vi "CreateTerminalVoltageDAQTask.vi"(8 "Error In":errorcluster) -> (0 "Error Out":errorcluster, 3 "Terminal Voltage Task":refnum<k21>)   [LabVIEW 2012]
uses:
  <vilib>/DAQmx/create/channels.llb/DAQmx Create Channel (AI-Voltage-Basic).vi
  <vilib>/DAQmx/configure/timing.llb/DAQmx Timing (Sample Clock).vi
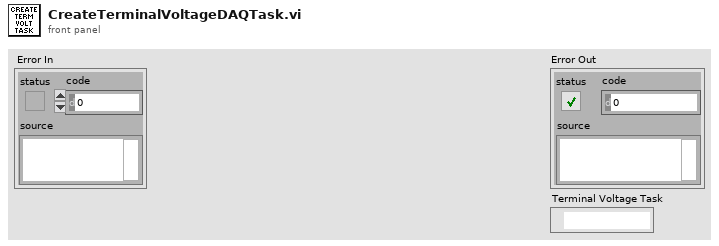
[diagram p1: front panel]
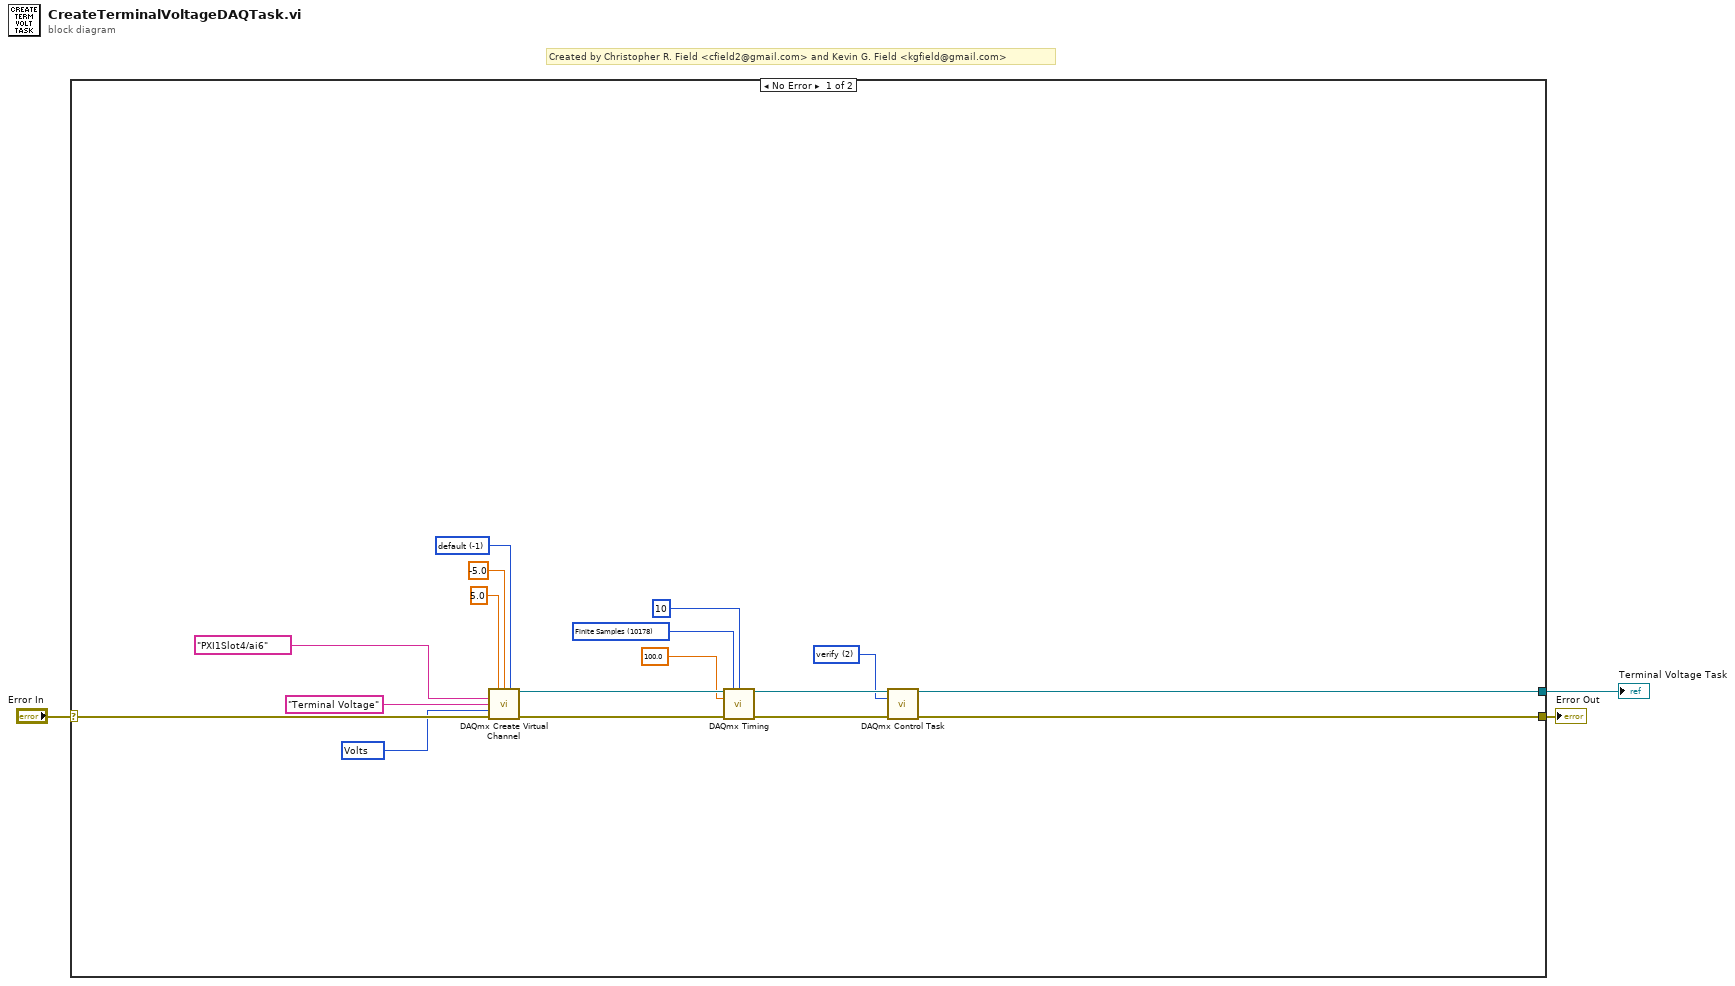
[diagram p0: block diagram]
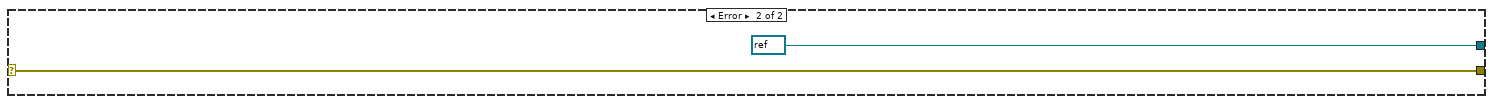
[diagram p2: hidden frame]
diagram:
  # "Created by Christopher R. Field <cfield2@gmail.com> and Kevin G. Field <kgfield@gmail.com>"
  n1 = case shown="No Error" "Error In" {
    selector: "Error In" -> [w20 w22]
    tunnel: [w19 w22] -> w2
    tunnel: [w18 refnum<k21> refnum ("task out")] -> w1
    frame No Error {
      w7 = -1 items=["default"=-1, "RSE"=10083, "NRSE"=10078, "Differential"=10106, "Pseudodifferential"=12529] ("input terminal configuration")
      w8 = 10348 items=["Volts"=10348, "From Custom Scale"=10065] ("units")
      w9 = 2 items=["verify"=2, "reserve"=4, "commit"=3, "unreserve"=5, "abort"=6] ("action")
      w13 = 10178 items=["Finite Samples"=10178, "Continuous Samples"=10123, "Hardware Timed Single Point"=12522] ("sample mode")
      n2 = call-poly <vilib>:"DAQmx Create Virtual Channel.vi"("maximum value"=5.0 ("minimum value"), "minimum value"=-5.0, "input terminal configuration"=w7, "physical channels"=tag "PXI1Slot4/ai6", "name to assign"="Terminal Voltage", "units"=w8, "error in"=w20) -> ("task out"=w17:refnum<k21>, "error out"=w16:errorcluster)  [unwired: 7 in]
      n3 = call-poly <vilib>:"DAQmx Timing.vi"("task/channels in"=w17, "sample mode"=w13, "samples per channel"=10, "rate"=100.0, "error in"=w16) -> ("task out"=w11:refnum<k21>, "error out"=w10:errorcluster)  [unwired: 9 in]
      n4 = call <vilib>:"DAQmx Control Task.vi"("task/channels in"=w11, "action"=w9, "error in"=w10) -> ("task out"=w18:refnum<k21>, "error out"=w19:errorcluster)  [unwired: 11 in]
    }
    frame Error {
    }
  }
  "Error Out" <- w2
  "Terminal Voltage Task" <- w1
